vi "Base Ctrl Set Obj Names.vi"() -> ()   [LabVIEW 2020]
uses:
  <vilib>/Utility/miscctls.llb/LVPointTypeDef.ctl
panel:
  out "Base Names":T1
  in  "Output Ports":string[](array[string])
  in  "Lamps":string[](array[string])
  in  "Turet Filter Names":string[](array[string])
  in  "Objecive Names":string[](array[string])
  out "Canceled":bool
  in  "Cancel":bool
  in  "Save":bool
  # "1"
  # "1"
  # "2"
  # "2"
  # "3"
  # "3"
  # "4"
  # "4"
  # "5"
  # "5"
  # "6"
  # "6"
  # "1"
  # "1"
  # "2"
  # "2"
  # "3"
  # "3"
  # "4"
  # "4"
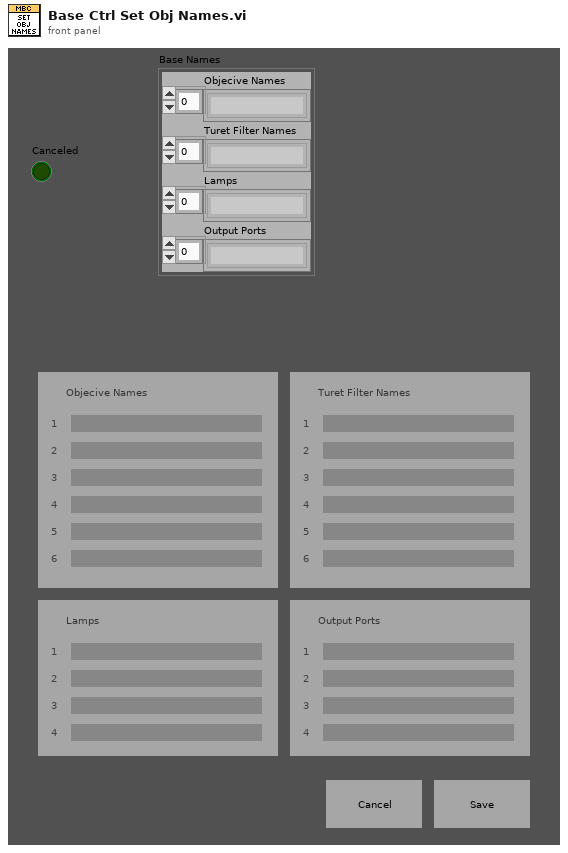
[diagram p1: front panel]
types:
  T1 = cluster{"Objecive Names":string[], "Turet Filter Names":string[], "Lamps":string[], "Output Ports":string[]}
  T2 = enum16{"Always On", "Always Off", "Off While Running"}
  T3 = typedef "LVPointTypeDef.ctl" = cluster{"Horizontal":i16, "Vertical":i16}
  T4 = typedef "LVBoundsTypeDef.ctl" = cluster{"Width":u32, "Height":u32}
  T5 = typedef "LVRectTypeDef.ctl" = cluster{"Left":i16, "Top":i16, "Right":i16, "Bottom":i16}
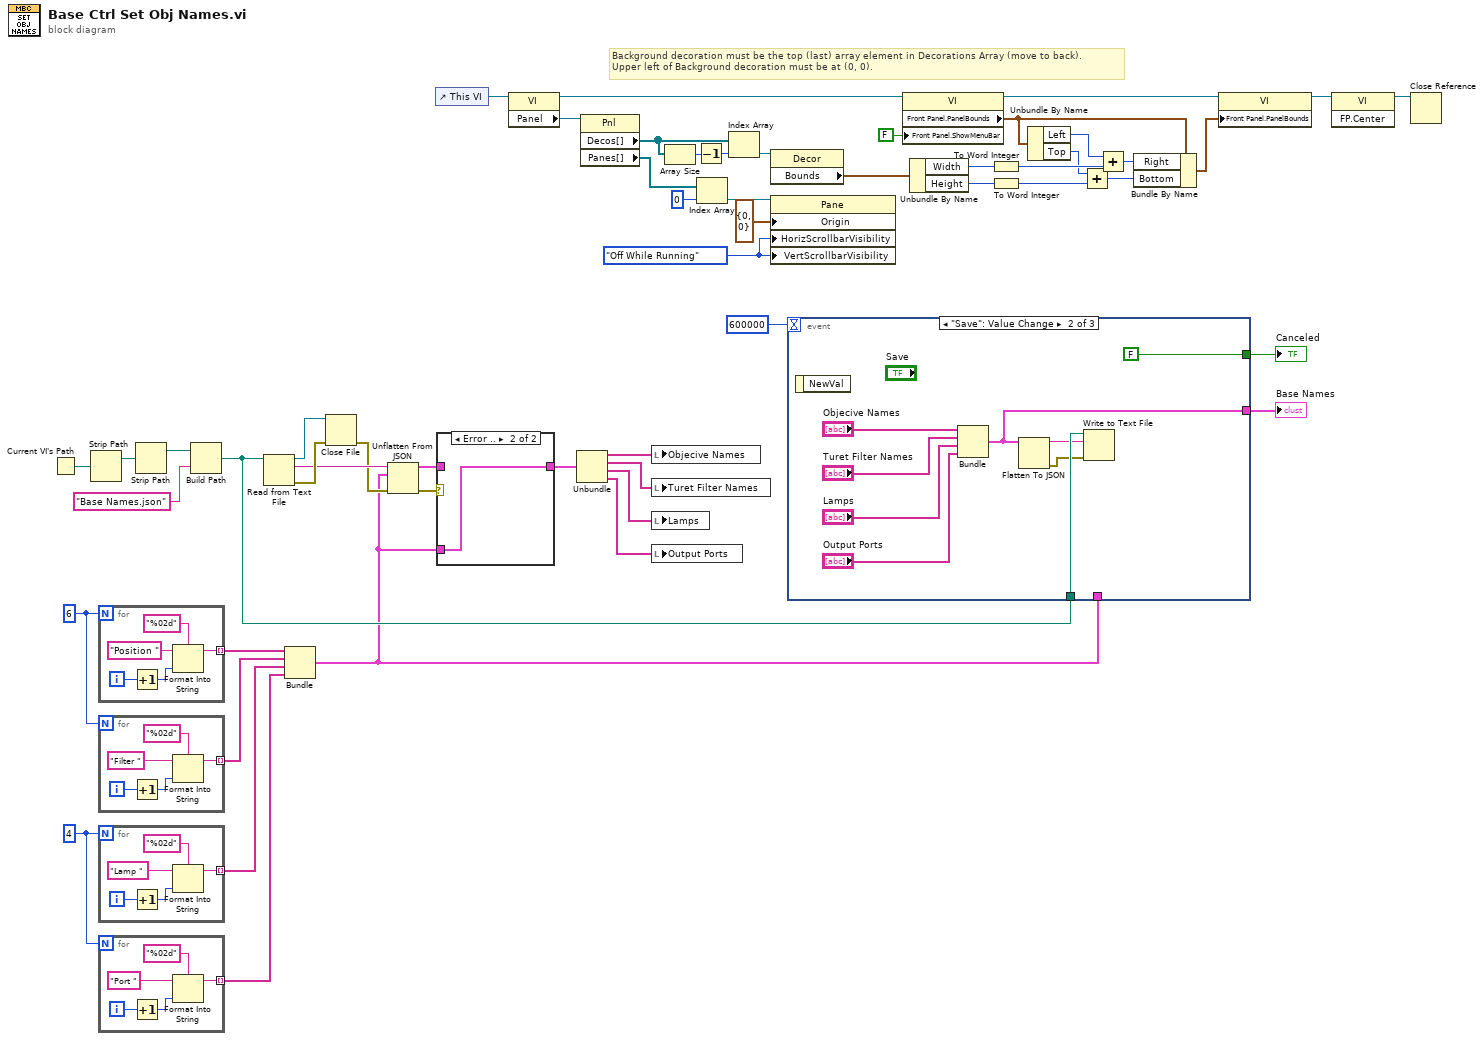
[diagram p0: block diagram]
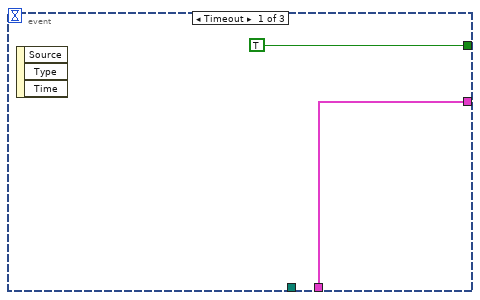
[diagram p3: hidden frame]
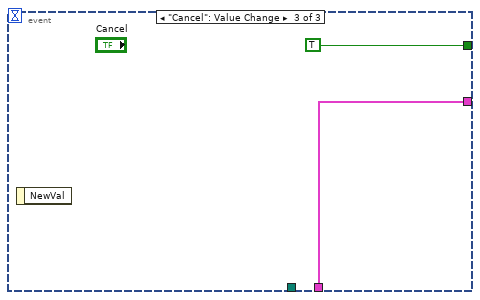
[diagram p4: hidden frame]
diagram:
  w12 = 4
  w13 = 6
  w44 = T2."Off While Running" ("Vertical Scrollbar Visibility")
  # "Background decoration must be the top (last) array element in Decorations Array (move to back).\nUpper left of Background decoration must be at (0, 0)."
  n1 = Current VI's Path() -> (path=w16:path)
  n2 = Strip Path(path=w16) -> (stripped path=w15:path)  [unwired: 1 out]
  n3 = for {
    N: w13 -> [_]
    tunnel: [w56] -> w11 mode=indexing
    i -> [w55]
    n4 = Increment(x=w55) -> (x+1=w54:i32)
    n5 = Format Into String(format string="%02d", initial string="Position ", w54) -> (resulting string=w56:string)  [unwired: 1 in, 1 out]
  }
  n6 = for {
    N: w13 -> [_]
    tunnel: [w61] -> w8 mode=indexing
    i -> [w60]
    n7 = Increment(x=w60) -> (x+1=w59:i32)
    n8 = Format Into String(format string="%02d", initial string="Filter ", w59) -> (resulting string=w61:string)  [unwired: 1 in, 1 out]
  }
  n9 = for {
    N: w12 -> [_]
    tunnel: [w66] -> w9 mode=indexing
    i -> [w65]
    n10 = Increment(x=w65) -> (x+1=w64:i32)
    n11 = Format Into String(format string="%02d", initial string="Lamp ", w64) -> (resulting string=w66:string)  [unwired: 1 in, 1 out]
  }
  n12 = for {
    N: w12 -> [_]
    tunnel: [w71] -> w10 mode=indexing
    i -> [w70]
    n13 = Increment(x=w70) -> (x+1=w69:i32)
    n14 = Format Into String(format string="%02d", initial string="Port ", w69) -> (resulting string=w71:string)  [unwired: 1 in, 1 out]
  }
  n15 = Strip Path(path=w15) -> (stripped path=w25:path)  [unwired: 1 out]
  n16 = Build Path(base path=w25, name or relative path="Base Names.json") -> (appended path=w14:path)
  n17 = Read from Text File(file (use dialog)=w14) -> (refnum out=w23:refnum<file>, text=w21:string, error out=w22:errorcluster)  [unwired: 3 in, 1 out]
  n18 = Bundle(w11, w8, w9, w10) -> (w2:cluster{string[], string[], string[], string[]})  [unwired: 1 in]
  n19 = Close File(refnum=w23, error in=w22) -> (error out=w20:errorcluster)  [unwired: 1 out]
  n20 = Unflatten From JSON(JSON string=w21, type and defaults=w2, error in (no error)=w20) -> (value=w18:cluster{string[], string[], string[], string[]}, error out=w19:errorcluster)  [unwired: 4 in]
  n21 = control-ref of="This VI"() -> (w30:refnum<vi>)
  n22 = case shown="Error .." w19 {
    tunnel: w18 -> [w74 _]
    tunnel: [w74 w75] -> w7
    tunnel: w2 -> [_ w75]
    frame No Error {
    }
    frame Error {
    }
  }
  n23 = property class="VI"(reference=w30) -> (reference out=w45:refnum<vi>, "Panel"=w38:refnum<vi>)  [unwired: 1 in, 1 out]
  n24 = Unbundle(w7) -> (w6:string[], w5:string[], w4:string[], w3:string[])
  n25 = property class="Pnl"(reference=w38) -> ("Decos[]"=w32:refnum<vi>[], "Panes[]"=w41:refnum<vi>[])  [unwired: 1 in, 2 out]
  n26 = local write "Objecive Names"(w6) -> ()
  n27 = local write "Turet Filter Names"(w5) -> ()
  n28 = local write "Lamps"(w4) -> ()
  n29 = local write "Output Ports"(w3) -> ()
  n30 = Array Size(array=w32) -> (size(s)=w37:i32)
  n31 = Decrement(x=w37) -> (x-1=w31:i32)
  n32 = Index Array(array=w41, index=0) -> (element=w40:refnum<vi>)
  n33 = Index Array(array=w32, index=w31) -> (element=w43:refnum<vi>)
  n34 = property class="Decor"(reference=w43) -> ("Bounds"=w46:T4)  [unwired: 1 in, 2 out]
  n35 = property class="Pane"(reference=w40, "Origin"=T3 {"Horizontal"=0, "Vertical"=0}, "HorizScrollbarVisibility"=w44, "VertScrollbarVisibility"=w44) -> ()  [unwired: 1 in, 2 out]
  n36 = event shown="[1] \"Save\": Value Change" {
    selector: _ -> [_ _ _]
    dyn-events: _ -> [_ _ _]
    timeout: 600000 -> [_ _ _]
    tunnel: w14 -> [_ w86 _]
    tunnel: [TRUE FALSE TRUE] -> w17
    tunnel: [w76 w78 w87] -> w1
    tunnel: w2 -> [w76 _ w87]
    event Timeout {
      n37 = event-data() -> ()  [unwired: 1 in, 3 out]
    }
    event "Save": Value Change {
      n38 = event-data() -> ()  [unwired: 1 in, 1 out]
      n39 = Bundle("Objecive Names"="Objecive Names", "Turet Filter Names"="Turet Filter Names", "Lamps"="Lamps", "Output Ports"="Output Ports") -> (w78:T1)  [unwired: 1 in]
      n40 = Flatten To JSON(anything=w78) -> (JSON string=w85:string, 11:w84:errorcluster)  [unwired: 2 in]
      n41 = Write to Text File(file (use dialog)=w86, text=w85, error in=w84) -> ()  [unwired: 1 in, 3 out]
    }
    event "Cancel": Value Change {
      n42 = event-data() -> ()  [unwired: 1 in, 1 out]
    }
  }
  "Canceled" <- w17
  "Base Names" <- w1
  n43 = property class="VI"(reference=w45, "Front Panel.ShowMenuBar"=FALSE ("Front Panel Window:Show Menu Bar")) -> (reference out=w47:refnum<vi>, "Front Panel.PanelBounds"=w48:T5)  [unwired: 1 in, 1 out]
  n44 = Unbundle By Name(w46) -> ("Width"=w51:u32, "Height"=w53:u32)
  n45 = To Word Integer(number=w51) -> (16bit integer=w52:i16)
  n46 = To Word Integer(number=w53) -> (16bit integer=w33:i16)
  n47 = Unbundle By Name(w48) -> ("Left"=w50:i16, "Top"=w35:i16)
  n48 = Add(x=w35, y=w33) -> (x+y=w34:i16)
  n49 = Add(x=w50, y=w52) -> (x+y=w36:i16)
  n50 = Bundle By Name(cluster=w48, "Right"=w36, "Bottom"=w34) -> (w49:T5)
  n51 = property class="VI"(reference=w47, "Front Panel.PanelBounds"=w49) -> (reference out=w27:refnum<vi>)  [unwired: 1 in, 1 out]
  n52 = invoke class="VI" method="FP.Center"(reference=w27) -> (reference out=w29:refnum<vi>)  [unwired: 2 in, 2 out]
  n53 = Close Reference(reference=w29) -> ()  [unwired: 1 in, 1 out]
